vi "test-runge-kutta-time-varying-solution.vi"(11 "T":dbl) -> (3 "output matrix":T1)   [LabVIEW 2019]
uses:
  <vilib>/Analysis/Matrix/Datatypes/RealMatrix.ctl
  <vilib>/Rock Robotics/WPI/ThirdParty/JAS_Junk/TrajLib/MatBuilder_Create.vi
  <vilib>/Rock Robotics/WPI/ThirdParty/JAS_Junk/TrajLib/Trajectory_Library.lvlib
  <vilib>/Analysis/Matrix/NI_Matrix.lvlib
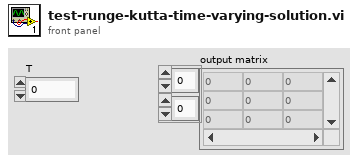
[diagram p1: front panel]
types:
  T1 = typedef "NI_Matrix.lvlib/RealMatrix.ctl" = dbl[][]
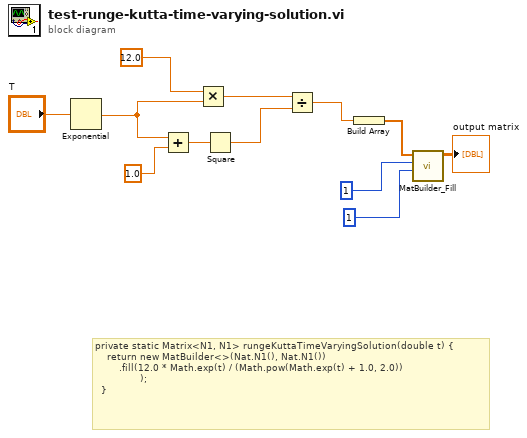
[diagram p0: block diagram]
diagram:
  # "private static Matrix<N1, N1> rungeKuttaTimeVaryingSolution(double t) {\n    return new MatBuilder<>(Nat.N1(), Nat.N1())\n        .fill(12.0 * Math.exp(t) / (Math.pow(Math.exp(t) + 1.0, 2.0))\n               );\n  }"
  n1 = Exponential(1:"T") -> (0:w8:dbl)
  n2 = Add(x=w8, y=1.0) -> (x+y=w6:dbl)
  n3 = Multiply(x=12.0, y=w8) -> (x*y=w5:dbl)
  n4 = Square(x=w6) -> (x^2=w4:dbl)
  n5 = Divide(x=w5, y=w4) -> (x/y=w3:dbl)
  n6 = Build Array(w3) -> (w2:dbl[])
  n7 = call <vilib>:"MatBuilder_Fill.vi"("Columns"=1, "Rows"=1, "Value List"=w2) -> ("output matrix"=→"output matrix":T1)  [unwired: 8 in]
